vi "SUMMER SUNDAY BYTE[Test].vi"() -> ()   [LabVIEW 2009]
uses:
  <vilib>/ULx/Create Channel.llb/ULx Create Channel (AI-Voltage-Basic).vi
  <vilib>/ULx/Create Channel.llb/ULx Create Channel (DO-Digital Output).vi
  <vilib>/ULx/Create Channel.llb/ULx Create Channel (DI-Digital Input).vi
  <vilib>/ULx/Read.llb/ULx Read (Analog DBL 1Chan 1Samp).vi
  <vilib>/ULx/Write.llb/ULx Write (Digital Bool 1Line 1Point).vi
  <vilib>/ULx/Read.llb/ULx Read (Digital 1D U8 NChan 1Samp).vi
panel:
  in  "Hutch Light":bool
  out "POWER":bool
  out "data":dbl format="%_6g"
  out "xray":bool caption="BitValue"
  out "ENERGY LEVEL":dbl(knob) scale=0.0..15.0
  out "Beam Pot":dbl format="%_6g"
  out "READY 2":bool
  out "DUMP":bool
  out "POWER":bool
  out "?":bool
  out "?":bool
  out "OPEN":bool
  out "CLOSED":bool
  out "READY":bool
  out "MAGNET FORCE":dbl(slide) scale=0.0..10.0
  out "READY":bool
  out "TEMPERATURE":dbl(slide) scale=0.0..100.0
  in  "stop":bool
  out "FAULT":bool
  out "POWER":bool
  out "FLOW IN GPM":dbl(knob) scale=0.0..15.0
  # "USERS LAB AREA"
  # "BEAM STATUS"
  # "ROOM"
  # "XRAY"
  # "PUMP STATION"
  # "MAGNET STATUS"
  # "ORBIT"
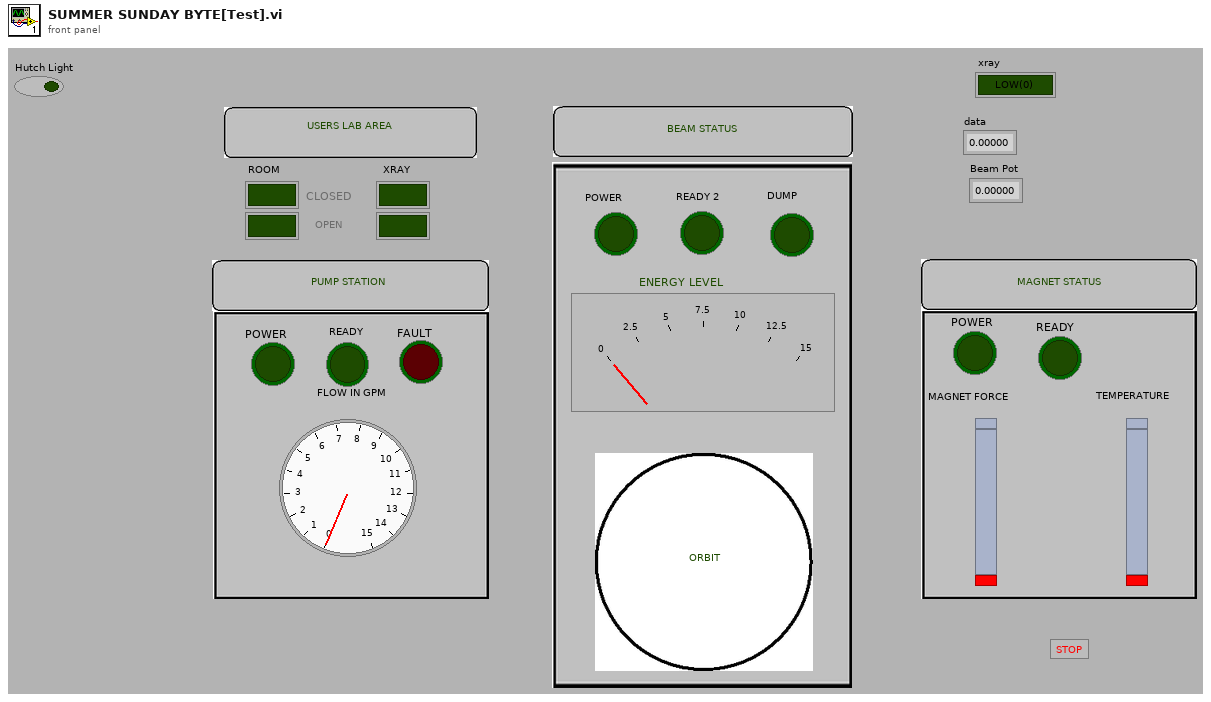
[diagram p1: front panel]
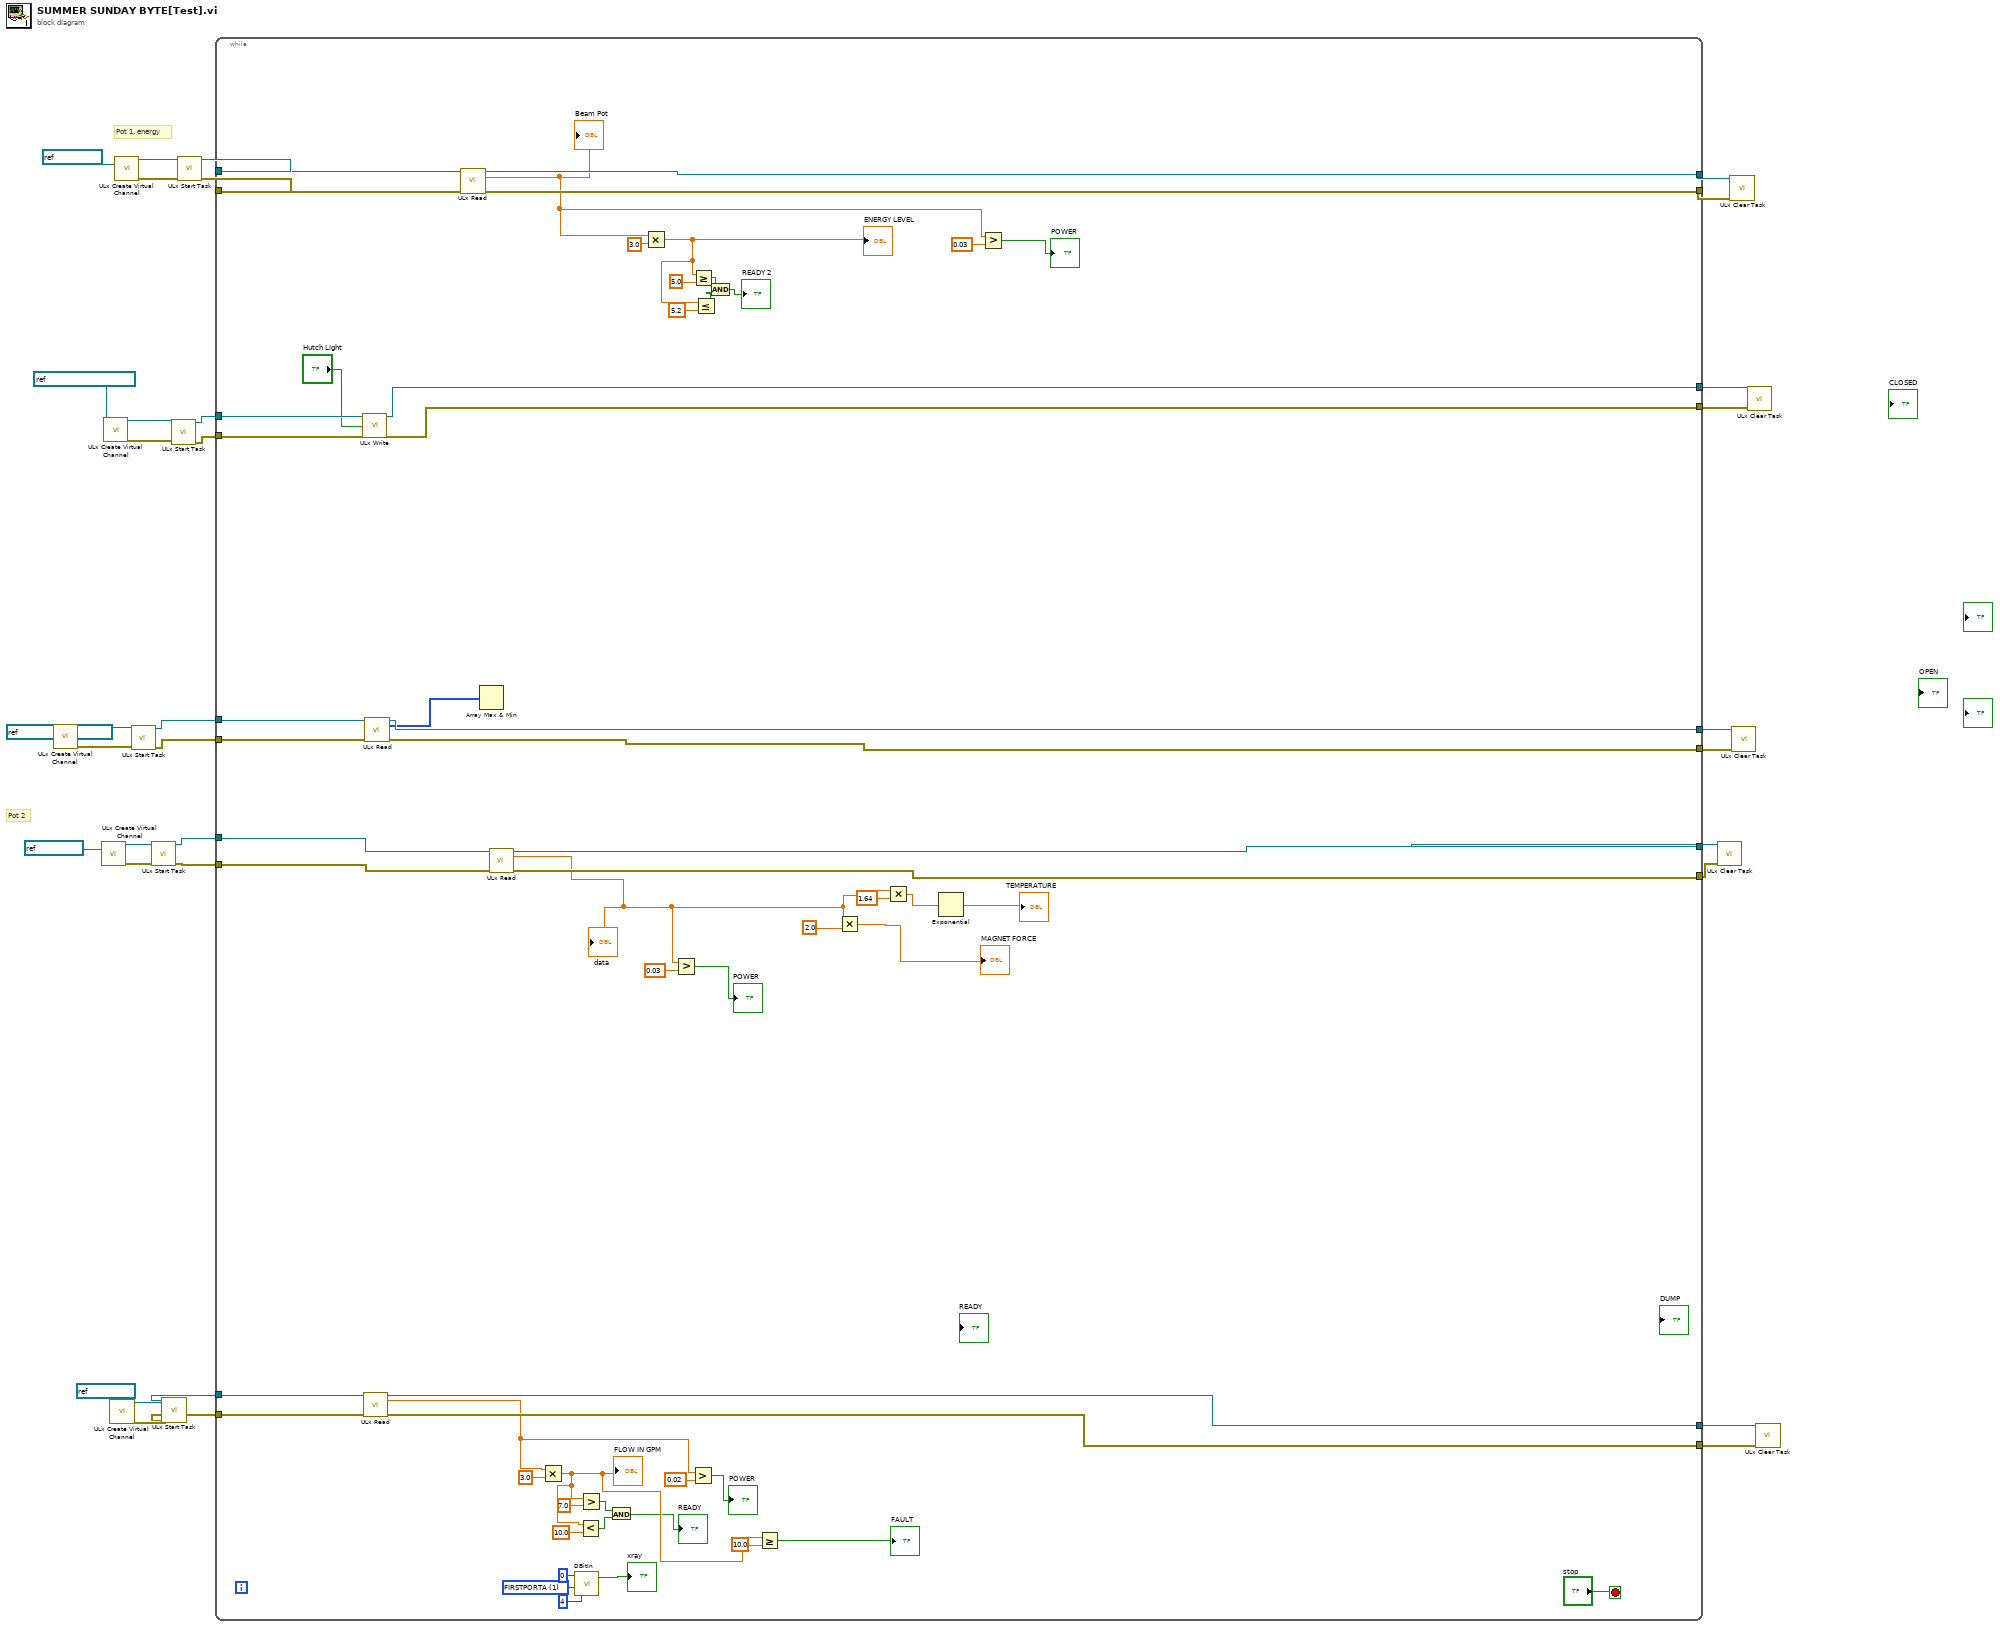
[diagram p0: block diagram]
diagram:
  # "Pot 2"
  # "Pot 1, energy"
  n1 = call-poly <vilib>:"ULx Create Virtual Channel.vi"("lines"=refnum<k21> "Dev0/1stPortA/Di0:7") -> ("task out"=w7:refnum<k24>, "error out"=w6:errorcluster)  [unwired: 13 in]
  n2 = call-poly <vilib>:"ULx Create Virtual Channel.vi"("physical channels"=refnum<k21> "Dev0/Ai1") -> ("task out"=w29:refnum<k24>, "error out"=w28:errorcluster)  [unwired: 13 in]
  n3 = call-poly <vilib>:"ULx Create Virtual Channel.vi"("lines"=refnum<k21> "Dev0/1stPortA/Do0") -> ("task out"=w14:refnum<k24>, "error out"=w13:errorcluster)  [unwired: 13 in]
  n4 = call-poly <vilib>:"ULx Create Virtual Channel.vi"("physical channels"=refnum<k21> "Dev0/Ai2") -> ("task out"=w21:refnum<k24>, "error out"=w20:errorcluster)  [unwired: 13 in]
  n5 = call-poly <vilib>:"ULx Create Virtual Channel.vi"("physical channels"=refnum<k21> "Dev0/Ai0") -> ("task out"=w35:refnum<k24>, "error out"=w34:errorcluster)  [unwired: 13 in]
  n6 = call <vilib>:"ULx Start Task.vi"("task in"=w7, "error in"=w6) -> ("task out"=w5:refnum<k24>, "error out"=w4:errorcluster)  [unwired: 12 in]
  n7 = call <vilib>:"ULx Start Task.vi"("task in"=w29, "error in"=w28) -> ("task out"=w27:refnum<k24>, "error out"=w26:errorcluster)  [unwired: 12 in]
  n8 = call <vilib>:"ULx Start Task.vi"("task in"=w21, "error in"=w20) -> ("task out"=w19:refnum<k24>, "error out"=w18:errorcluster)  [unwired: 12 in]
  n9 = call <vilib>:"ULx Start Task.vi"("task in"=w14, "error in"=w13) -> ("task out"=w11:refnum<k24>, "error out"=w10:errorcluster)  [unwired: 12 in]
  n10 = call <vilib>:"ULx Start Task.vi"("task in"=w35, "error in"=w34) -> ("task out"=w33:refnum<k24>, "error out"=w32:errorcluster)  [unwired: 12 in]
  n11 = while {
    tunnel: w33 -> [w91]
    tunnel: w32 -> [w90]
    tunnel: [w89] -> w31
    tunnel: [w88] -> w30
    tunnel: w27 -> [w86]
    tunnel: w26 -> [w85]
    tunnel: [w84] -> w25
    tunnel: [w83] -> w24
    tunnel: w19 -> [w80]
    tunnel: w18 -> [w79]
    tunnel: [w78] -> w16
    tunnel: [w77] -> w15
    tunnel: w11 -> [w46]
    tunnel: w10 -> [w45]
    tunnel: [w44] -> w9
    tunnel: [w43] -> w8
    tunnel: w5 -> [w41]
    tunnel: w4 -> [w40]
    tunnel: [w39] -> w2
    tunnel: [w37] -> w1
    stop <- "stop" stop-if-true
    w75 = 1 items=["AUXPORT", "FIRSTPORTA"] ("PortType")
    n12 = call-poly <vilib>:"ULx Write.vi"("task in"=w46, "data"="Hutch Light", "error in"=w45) -> ("task out"=w44:refnum<k24>, "error out"=w43:errorcluster)  [unwired: 10 in, 1 out]
    n13 = call-poly <vilib>:"ULx Read.vi"("task in"=w80, "error in"=w79) -> ("task out"=w78:refnum<k24>, "data"=w67:dbl, "error out"=w77:errorcluster)  [unwired: 11 in]
    n14 = call-poly <vilib>:"ULx Read.vi"("task in"=w41, "error in"=w40) -> ("task out"=w37:refnum<k24>, "data"=w36:u8[], "error out"=w39:errorcluster)  [unwired: 11 in]
    n15 = call-poly <vilib>:"ULx Read.vi"("task in"=w91, "error in"=w90) -> ("task out"=w89:refnum<k24>, "data"=w47:dbl, "error out"=w88:errorcluster)  [unwired: 11 in]
    "Beam Pot" <- w47
    n16 = Array Max & Min(array=w36) -> ()  [unwired: 4 out]
    n17 = call-poly <vilib>:"ULx Read.vi"("task in"=w86, "error in"=w85) -> ("task out"=w84:refnum<k24>, "data"=w51:dbl, "error out"=w83:errorcluster)  [unwired: 11 in]
    "data" <- w51
    n18 = Multiply(x=w67, y=3.0) -> (x*y=w55:dbl)
    "FLOW IN GPM" <- w55
    n19 = call <menus>:"DBitIn.VI"("BitNum"=4, "PortType"=w75, "BoardNum"=u32 0) -> ("BitValue"=→"xray":bool)  [unwired: 1 out]
    n20 = Less?(x=w55, y=10.0) -> (x < y?=w53:bool)
    n21 = Greater?(x=w55, y=7.0) -> (0:w54:bool)
    n22 = And(x=w54, y=w53) -> (x .and. y?=→"READY":bool)
    n23 = Multiply(x=w47, y=3.0) -> (x*y=w64:dbl)
    "ENERGY LEVEL" <- w64
    n24 = Greater?(x=w51, y=0.03) -> (0:→"POWER":bool)
    n25 = Greater?(x=w67, y=0.02) -> (0:→"POWER":bool)
    n26 = Greater Or Equal?(x=w64, y=5.0) -> (x >= y?=w61:bool)
    n27 = Less Or Equal?(x=w64, y=5.2) -> (x <= y?=w60:bool)
    n28 = And(x=w61, y=w60) -> (x .and. y?=→"READY 2":bool)
    n29 = Greater Or Equal?(x=w55, y=10.0) -> (x >= y?=→"FAULT":bool)
    n30 = Multiply(x=w51, y=2.0) -> (x*y=→"MAGNET FORCE":dbl)
    n31 = Multiply(x=w51, y=1.64) -> (x*y=w49:dbl)
    n32 = Exponential(1:w49) -> (0:→"TEMPERATURE":dbl)
    n33 = Greater?(x=w47, y=0.03) -> (0:→"POWER":bool)
  }
  n34 = call <vilib>:"ULx Clear Task.vi"("task in"=w25, "error in"=w24) -> ()  [unwired: 13 in, 1 out]
  n35 = call <vilib>:"ULx Clear Task.vi"("task in"=w31, "error in"=w30) -> ()  [unwired: 13 in, 1 out]
  n36 = call <vilib>:"ULx Clear Task.vi"("task in"=w1, "error in"=w2) -> ()  [unwired: 13 in, 1 out]
  n37 = call <vilib>:"ULx Clear Task.vi"("task in"=w9, "error in"=w8) -> ()  [unwired: 13 in, 1 out]
  n38 = call <vilib>:"ULx Clear Task.vi"("task in"=w16, "error in"=w15) -> ()  [unwired: 13 in, 1 out]
